vi "System_Configuration_Set.vi"(3 "error in (no error)":errorcluster, 4 "Device Selection":T1, 5 "Devices":T3, 6 "Config":T2 {"Compute Config"."Post-Trigger Time" format="%.3f ms"; "Compute Config"."Pre-Trigger Time" format="%.3f ms"; "Compute Config"."Trigger Frequency" items=["Single", "Continuous"]; "Compute Config"."Trigger Type" items=["GPS Time", "Anomaly Detection"]; "SDR Config"."WRx 2\nGain Attenuation" min=0 max=27 step=1 scale=0.0..27.0; "SDR Config"."WRx 2\nRSSI Threshold" format="%.2f dBm"; "SDR Config"."WRx 2\nGain Mode" items=["Automatic", "Fixed"]; "SDR Config"."WRx 2\nBandwidth Mode" items=["500 MHz"]; "SDR Config"."WRx 2\nIF Frequency" items=["1200 MHz", "1400 MHz", "3000 MHZ"]; "SDR Config"."WRx 1\nGain Attenuation" min=0 max=27 step=1 scale=0.0..27.0; "SDR Config"."WRx 1\nRSSI Threshold" format="%.2f dBm"; "SDR Config"."WRx 1\nGain Mode" items=["Automatic", "Fixed"]; "SDR Config"."WRx 1\nBandwidth Mode" items=["500 MHz"]; "SDR Config"."WRx 1\nIF Frequency" items=["1200 MHz", "1400 MHz", "3000 MHZ"]}) -> ()   [LabVIEW 2024]
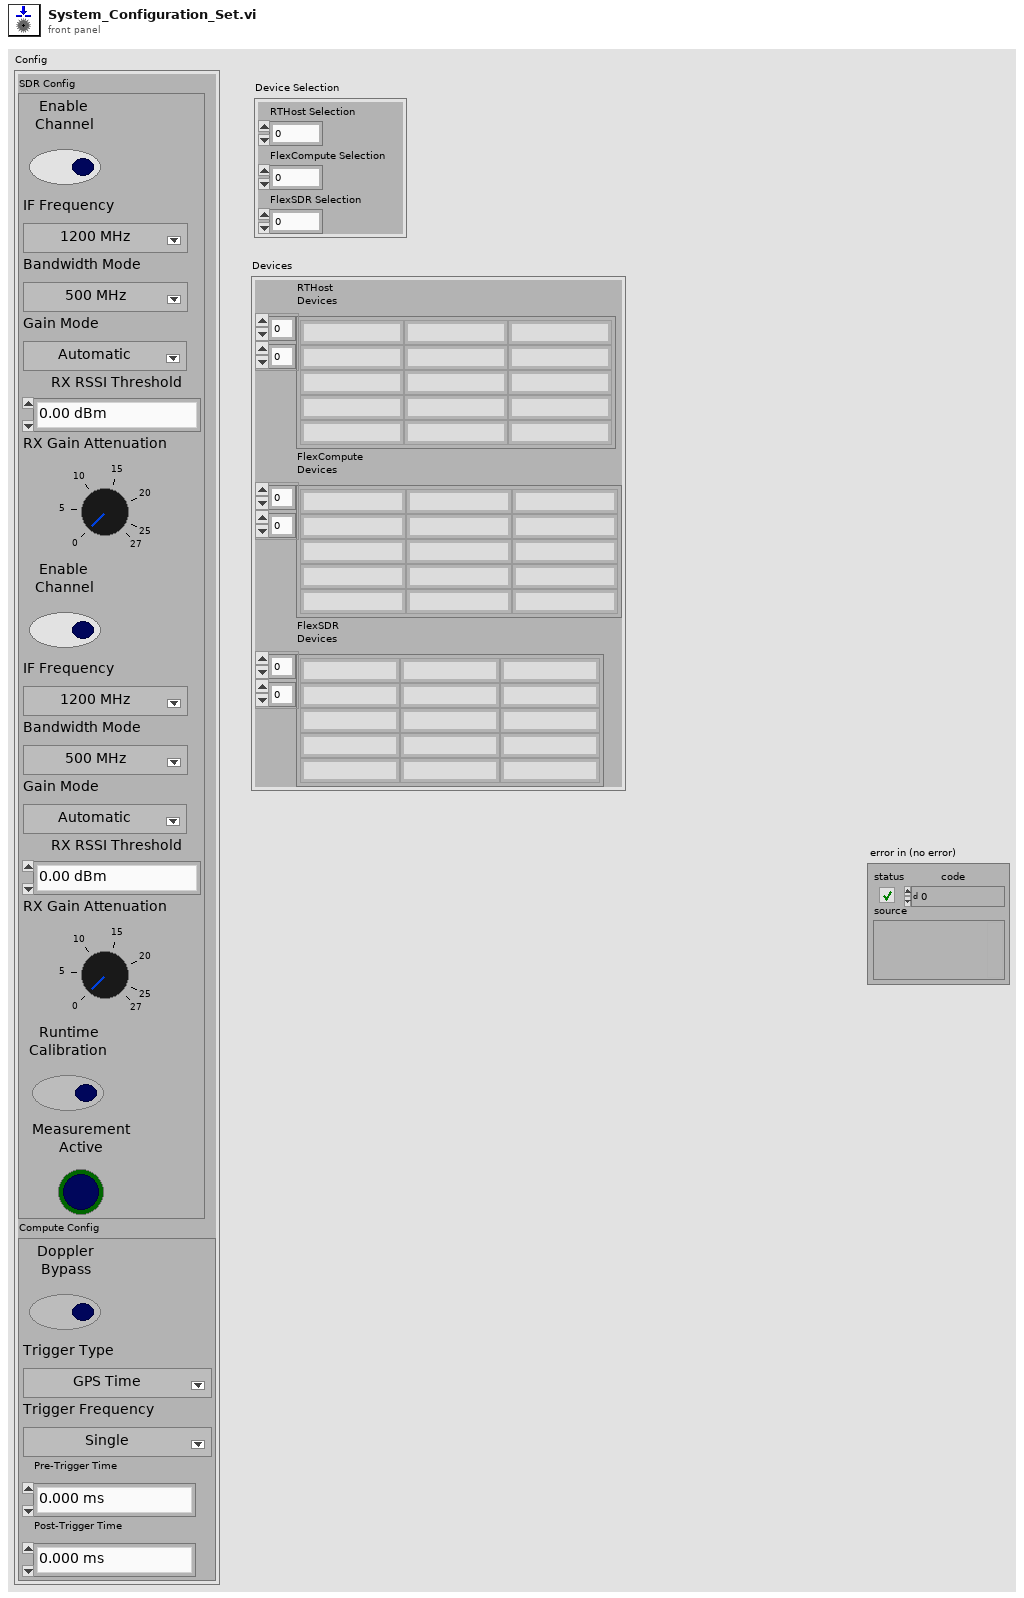
[diagram p1: front panel]
types:
  T1 = cluster{"RTHost Selection":u16, "FlexCompute Selection":u16, "FlexSDR Selection":u16}
  T2 = cluster{"SDR Config":cluster{"WRx 1\nEnable Channel":bool, "WRx 1\nIF Frequency":u16, "WRx 1\nBandwidth Mode":u16, "WRx 1\nGain Mode":u16, "WRx 1\nRSSI Threshold":dbl, "WRx 1\nGain Attenuation":i64, "WRx 2\nEnable Channel":bool, "WRx 2\nIF Frequency":u16, "WRx 2\nBandwidth Mode":u16, "WRx 2\nGain Mode":u16, "WRx 2\nRSSI Threshold":dbl, "WRx 2\nGain Attenuation":i64, "Runtime\nCalibration":bool, "Measurement\nActive":bool}, "Compute Config":cluster{"Doppler\nBypass":bool, "Trigger Type":u16, "Trigger Frequency":u16, "Pre-Trigger Time":dbl, "Post-Trigger Time":dbl}}
  T3 = cluster{"RTHost\nDevices":string[][], "FlexCompute\nDevices":string[][], "FlexSDR\nDevices":string[][]}
  T4 = cluster{"WRx 1\nEnable Channel":bool, "WRx 1\nIF Frequency":u16, "WRx 1\nBandwidth Mode":u16, "WRx 1\nGain Mode":u16, "WRx 1\nRSSI Threshold":dbl, "WRx 1\nGain Attenuation":i64, "WRx 2\nEnable Channel":bool, "WRx 2\nIF Frequency":u16, "WRx 2\nBandwidth Mode":u16, "WRx 2\nGain Mode":u16, "WRx 2\nRSSI Threshold":dbl, "WRx 2\nGain Attenuation":i64, "Runtime\nCalibration":bool, "Measurement\nActive":bool}
  T5 = enum16{"open", "replace", "create", "open or create", "replace or create", "replace or create with confirmation"}
  T6 = cluster{"Doppler\nBypass":bool, "Trigger Type":u16, "Trigger Frequency":u16, "Pre-Trigger Time":dbl, "Post-Trigger Time":dbl}
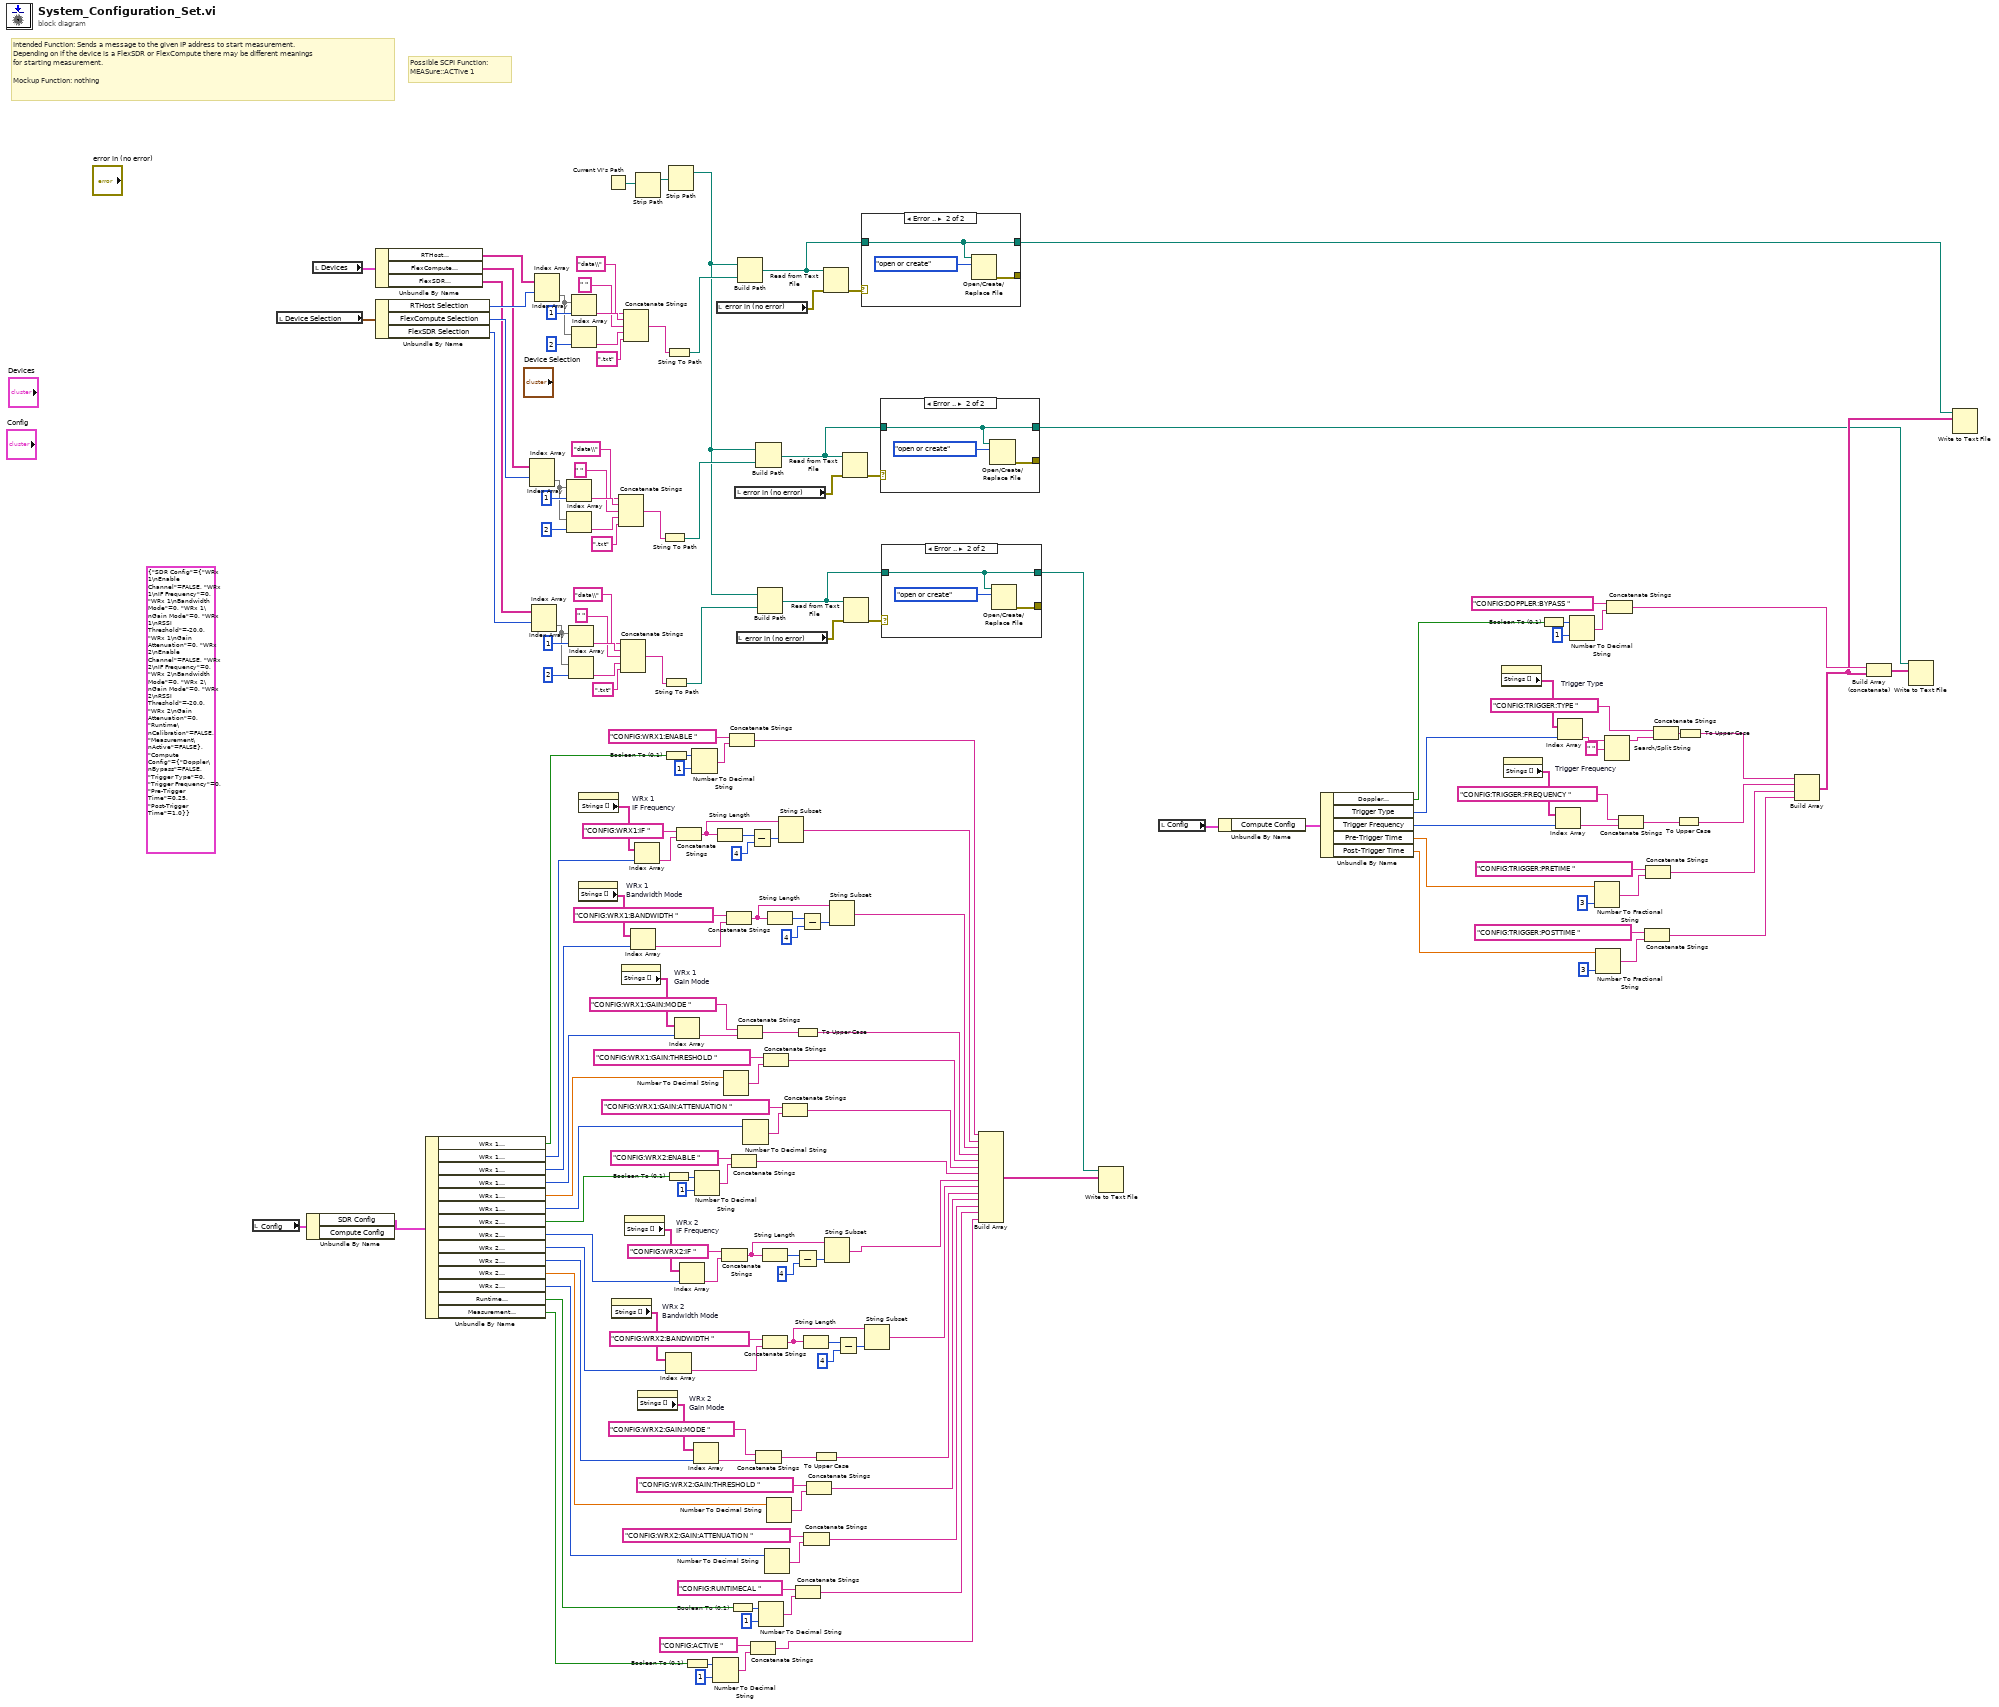
[diagram p0: block diagram]
diagram:
  (unwired) T2 {"SDR Config"={"WRx 1\nEnable Channel"=FALSE, "WRx 1\nIF Frequency"=0, "WRx 1\nBandwidth Mode"=0, "WRx 1\nGain Mode"=0, "WRx 1\nRSSI Threshold"=-20.0, "WRx 1\nGain Attenuation"=0, "WRx 2\nEnable Channel"=FALSE, "WRx 2\nIF Frequency"=0, "WRx 2\nBandwidth Mode"=0, "WRx 2\nGain Mode"=0, "WRx 2\nRSSI Threshold"=-20.0, "WRx 2\nGain Attenuation"=0, "Runtime\nCalibration"=FALSE, "Measurement\nActive"=FALSE}, "Compute Config"={"Doppler\nBypass"=FALSE, "Trigger Type"=0, "Trigger Frequency"=0, "Pre-Trigger Time"=0.25, "Post-Trigger Time"=1.0}} ("Config 2")
  # "Possible SCPI Function:\nMEASure::ACTive 1"
  # "Intended Function: Sends a message to the given IP address to start measurement.\nDepending on if the device is a FlexSDR or FlexCompute there may be different meanings\nfor starting measurement.\n\nMockup Function: nothing"
  n1 = local read "Config"() -> (w113:T2)
  n2 = local read "Device Selection"() -> (w147:T1)
  n3 = Unbundle By Name(w113) -> ("SDR Config"=w111:T4)  [unwired: 1 out]
  n4 = local read "Devices"() -> (w167:T3)
  n5 = Unbundle By Name(w167) -> ("RTHost\nDevices"=w146:string[][], "FlexCompute\nDevices"=w131:string[][], "FlexSDR\nDevices"=w115:string[][])
  n6 = Unbundle By Name(w147) -> ("RTHost Selection"=w145:u16, "FlexCompute Selection"=w130:u16, "FlexSDR Selection"=w114:u16)
  n7 = Unbundle By Name(w111) -> ("WRx 1\nEnable Channel"=w110:bool, "WRx 1\nIF Frequency"=w109:u16, "WRx 1\nBandwidth Mode"=w100:u16, "WRx 1\nGain Mode"=w98:u16, "WRx 1\nRSSI Threshold"=w97:dbl, "WRx 1\nGain Attenuation"=w93:i64, "WRx 2\nEnable Channel"=w54:bool, "WRx 2\nIF Frequency"=w53:u16, "WRx 2\nBandwidth Mode"=w65:u16, "WRx 2\nGain Mode"=w73:u16, "WRx 2\nRSSI Threshold"=w79:dbl, "WRx 2\nGain Attenuation"=w80:i64, "Runtime\nCalibration"=w83:bool, "Measurement\nActive"=w88:bool)
  n8 = Index Array(array=w131, index (row)=w130) -> (element=w143:string[])  [unwired: 1 in]
  n9 = Index Array(array=w115, index (row)=w114) -> (element=w128:string[])  [unwired: 1 in]
  n10 = Index Array(array=w146, index (row)=w145) -> (element=w176:string[])  [unwired: 1 in]
  n11 = Index Array(array=w143, index=1) -> (element=w141:string)
  n12 = Index Array(array=w143, index=2) -> (element=w140:string)
  n13 = Index Array(array=w128, index=1) -> (element=w126:string)
  n14 = Index Array(array=w128, index=2) -> (element=w125:string)
  n15 = Index Array(array=w176, index=1) -> (element=w174:string)
  n16 = Index Array(array=w176, index=2) -> (element=w173:string)
  n17 = property on="WRx 1\nBandwidth Mode" class="Ring (strict)"() -> ("Strings []"=w101:string[])  [unwired: 2 in, 2 out]
  n18 = property on="WRx 1\nIF Frequency" class="Ring (strict)"() -> ("Strings []"=w108:string[])  [unwired: 2 in, 2 out]
  n19 = Current VI's Path() -> (path=w178:path)
  n20 = property on="WRx 2\nBandwidth Mode" class="Ring (strict)"() -> ("Strings []"=w64:string[])  [unwired: 2 in, 2 out]
  n21 = Concatenate Strings("data\\" ("string"), w141, " " ("element"), w140, ".txt" ("string")) -> (w136:string)
  n22 = Concatenate Strings("data\\" ("string"), w126, " " ("element"), w125, ".txt" ("string")) -> (w121:string)
  n23 = property on="WRx 1\nGain Mode" class="Ring (strict)"() -> ("Strings []"=w99:string[])  [unwired: 2 in, 2 out]
  n24 = Concatenate Strings("data\\" ("string"), w174, " " ("element"), w173, ".txt" ("string")) -> (w169:string)
  n25 = property on="WRx 2\nIF Frequency" class="Ring (strict)"() -> ("Strings []"=w52:string[])  [unwired: 2 in, 2 out]
  n26 = Index Array(array=w101, index=w100) -> (element=w107:string)
  n27 = Index Array(array=w108, index=w109) -> (element=w161:string)
  n28 = Strip Path(path=w178) -> (stripped path=w163:path)  [unwired: 1 out]
  n29 = property on="WRx 2\nGain Mode" class="Ring (strict)"() -> ("Strings []"=w72:string[])  [unwired: 2 in, 2 out]
  n30 = String To Path(string=w136) -> (path=w135:path)
  n31 = String To Path(string=w121) -> (path=w120:path)
  n32 = Boolean To (0,1)(Boolean=w110) -> (0, 1=w159:i16)
  n33 = Boolean To (0,1)(Boolean=w54) -> (0, 1=w57:i16)
  n34 = Index Array(array=w64, index=w65) -> (element=w71:string)
  n35 = String To Path(string=w169) -> (path=w168:path)
  n36 = Strip Path(path=w163) -> (stripped path=w116:path)  [unwired: 1 out]
  n37 = Index Array(array=w99, index=w98) -> (element=w151:string)
  n38 = Concatenate Strings("CONFIG:WRX1:IF " ("string"), w161) -> (w152:string)
  n39 = Index Array(array=w52, index=w53) -> (element=w37:string)
  n40 = Boolean To (0,1)(Boolean=w88) -> (0, 1=w91:i16)
  n41 = Number To Decimal String(number=w159, width (-)=i16 1) -> (decimal integer string=w160:string)
  n42 = Index Array(array=w72, index=w73) -> (element=w76:string)
  n43 = Number To Decimal String(number=w57, width (-)=i16 1) -> (decimal integer string=w58:string)
  n44 = Number To Decimal String(number=w91, width (-)=i16 1) -> (decimal integer string=w92:string)
  n45 = local read "error in (no error)"() -> (w166:errorcluster)
  n46 = String Length(string=w152) -> (length=w155:i32)
  n47 = Concatenate Strings("CONFIG:WRX2:IF " ("string"), w37) -> (w59:string)
  n48 = Number To Decimal String(number=w97) -> (decimal integer string=w96:string)  [unwired: 1 in]
  n49 = Concatenate Strings("CONFIG:WRX1:BANDWIDTH " ("string"), w107) -> (w102:string)
  n50 = Concatenate Strings("CONFIG:WRX1:ENABLE " ("string"), w160) -> (w51:string)
  n51 = Boolean To (0,1)(Boolean=w83) -> (0, 1=w86:i16)
  n52 = Concatenate Strings("CONFIG:WRX2:ENABLE " ("string"), w58) -> (w45:string)
  n53 = local read "error in (no error)"() -> (w134:errorcluster)
  n54 = local read "error in (no error)"() -> (w119:errorcluster)
  n55 = Build Path(base path=w116, name or relative path=w168) -> (appended path=w164:path)
  n56 = Concatenate Strings("CONFIG:WRX1:GAIN:MODE " ("string"), w151) -> (w149:string)
  n57 = Number To Decimal String(number=w93) -> (decimal integer string=w94:string)  [unwired: 1 in]
  n58 = Subtract(x=w155, y=4) -> (x-y=w153:i32)
  n59 = Concatenate Strings("CONFIG:ACTIVE " ("string"), w92) -> (w44:string)
  n60 = Build Path(base path=w116, name or relative path=w135) -> (appended path=w132:path)
  n61 = Concatenate Strings("CONFIG:WRX2:GAIN:MODE " ("string"), w76) -> (w74:string)
  n62 = Build Path(base path=w116, name or relative path=w120) -> (appended path=w117:path)
  n63 = Number To Decimal String(number=w86, width (-)=i16 1) -> (decimal integer string=w87:string)
  n64 = String Length(string=w59) -> (length=w62:i32)
  n65 = Concatenate Strings("CONFIG:WRX2:BANDWIDTH " ("string"), w71) -> (w66:string)
  n66 = Concatenate Strings("CONFIG:WRX1:GAIN:THRESHOLD " ("string"), w96) -> (w47:string)
  n67 = Number To Decimal String(number=w80) -> (decimal integer string=w81:string)  [unwired: 1 in]
  n68 = Number To Decimal String(number=w79) -> (decimal integer string=w78:string)  [unwired: 1 in]
  n69 = String Length(string=w102) -> (length=w105:i32)
  n70 = String Subset(string=w152, length (rest)=w153) -> (substring=w50:string)  [unwired: 1 in]
  n71 = Concatenate Strings("CONFIG:WRX1:GAIN:ATTENUATION " ("string"), w94) -> (w46:string)
  n72 = To Upper Case(1:w149) -> (0:w48:string)
  n73 = Subtract(x=w62, y=4) -> (x-y=w60:i32)
  n74 = Concatenate Strings("CONFIG:RUNTIMECAL " ("string"), w87) -> (w43:string)
  n75 = Subtract(x=w105, y=4) -> (x-y=w103:i32)
  n76 = String Length(string=w66) -> (length=w69:i32)
  n77 = Concatenate Strings("CONFIG:WRX2:GAIN:ATTENUATION " ("string"), w81) -> (w42:string)
  n78 = Concatenate Strings("CONFIG:WRX2:GAIN:THRESHOLD " ("string"), w78) -> (w41:string)
  n79 = To Upper Case(1:w74) -> (0:w40:string)
  n80 = Read from Text File(file (use dialog)=w164, error in=w166) -> (error out=w165:errorcluster)  [unwired: 2 in, 3 out]
  n81 = String Subset(string=w59, length (rest)=w60) -> (substring=w38:string)  [unwired: 1 in]
  n82 = String Subset(string=w102, length (rest)=w103) -> (substring=w49:string)  [unwired: 1 in]
  n83 = Subtract(x=w69, y=4) -> (x-y=w67:i32)
  n84 = Read from Text File(file (use dialog)=w132, error in=w134) -> (error out=w133:errorcluster)  [unwired: 2 in, 3 out]
  n85 = Read from Text File(file (use dialog)=w117, error in=w119) -> (error out=w118:errorcluster)  [unwired: 2 in, 3 out]
  n86 = case shown="Error .." w165 {
    selector: w165 -> [w179 _]
    tunnel: w164 -> [w180 w182]
    tunnel: [w180 w182] -> w14
    tunnel: [w179 w181] -> _
    frame No Error {
    }
    frame Error {
      n87 = Open/Create/Replace File(file path (use dialog)=w182, operation (0:open)=T5."open or create") -> (error out=w181:errorcluster)  [unwired: 4 in, 2 out]
    }
  }
  n88 = String Subset(string=w66, length (rest)=w67) -> (substring=w39:string)  [unwired: 1 in]
  n89 = case shown="Error .." w133 {
    selector: w133 -> [w184 _]
    tunnel: w132 -> [w185 w187]
    tunnel: [w185 w187] -> w12
    tunnel: [w184 w186] -> _
    frame No Error {
    }
    frame Error {
      n90 = Open/Create/Replace File(file path (use dialog)=w187, operation (0:open)=T5."open or create") -> (error out=w186:errorcluster)  [unwired: 4 in, 2 out]
    }
  }
  n91 = case shown="Error .." w118 {
    selector: w118 -> [w189 _]
    tunnel: w117 -> [w190 w192]
    tunnel: [w190 w192] -> w112
    tunnel: [w189 w191] -> _
    frame No Error {
    }
    frame Error {
      n92 = Open/Create/Replace File(file path (use dialog)=w192, operation (0:open)=T5."open or create") -> (error out=w191:errorcluster)  [unwired: 4 in, 2 out]
    }
  }
  n93 = Build Array(w51, w50, w49, w48, w47, w46, w45, w38, w39, w40, w41, w42, w43, w44) -> (w162:string[])
  n94 = Write to Text File(file (use dialog)=w112, text=w162) -> ()  [unwired: 2 in, 3 out]
  n95 = local read "Config"() -> (w36:T2)
  n96 = Unbundle By Name(w36) -> ("Compute Config"=w35:T6)
  n97 = Unbundle By Name(w35) -> ("Doppler\nBypass"=w30:bool, "Trigger Type"=w26:u16, "Trigger Frequency"=w21:u16, "Pre-Trigger Time"=w7:dbl, "Post-Trigger Time"=w9:dbl)
  n98 = property on="Trigger Type" class="Ring (strict)"() -> ("Strings []"=w27:string[])  [unwired: 2 in, 2 out]
  n99 = property on="Trigger Frequency" class="Ring (strict)"() -> ("Strings []"=w22:string[])  [unwired: 2 in, 2 out]
  n100 = Boolean To (0,1)(Boolean=w30) -> (0, 1=w33:i16)
  n101 = Index Array(array=w22, index=w21) -> (element=w25:string)
  n102 = Index Array(array=w27, index=w26) -> (element=w3:string)
  n103 = Number To Decimal String(number=w33, width (-)=i16 1) -> (decimal integer string=w34:string)
  n104 = Number To Fractional String(number=w7, precision (6)=i16 3) -> (F-format string=w6:string)  [unwired: 2 in]
  n105 = Number To Fractional String(number=w9, precision (6)=i16 3) -> (F-format string=w8:string)  [unwired: 2 in]
  n106 = Search/Split String(string=w3, search string/char (-)=" ") -> (substring before match=w1:string)  [unwired: 1 in, 2 out]
  n107 = Concatenate Strings("CONFIG:DOPPLER:BYPASS " ("string"), w34) -> (w16:string)
  n108 = Concatenate Strings("CONFIG:TRIGGER:FREQUENCY " ("string"), w25) -> (w23:string)
  n109 = Concatenate Strings("CONFIG:TRIGGER:POSTTIME " ("string"), w8) -> (w17:string)
  n110 = Concatenate Strings("CONFIG:TRIGGER:PRETIME " ("string"), w6) -> (w18:string)
  n111 = Concatenate Strings("CONFIG:TRIGGER:TYPE " ("string"), w1) -> (w28:string)
  n112 = To Upper Case(1:w23) -> (0:w19:string)
  n113 = To Upper Case(1:w28) -> (0:w20:string)
  n114 = Build Array(w20, w19, w18, w17) -> (w15:string[])
  n115 = Build Array (concatenate)(w16, w15) -> (w13:string[])
  n116 = Write to Text File(file (use dialog)=w12, text=w13) -> ()  [unwired: 2 in, 3 out]
  n117 = Write to Text File(file (use dialog)=w14, text=w15) -> ()  [unwired: 2 in, 3 out]
